vi "Debug.vi"(11 "Msg In":string) -> (3 "Array - String":string[](array[string]))   [LabVIEW 2014, in "Controller.lvlib" / "Controller.lvclass"]
uses:
  Controller.lvclass
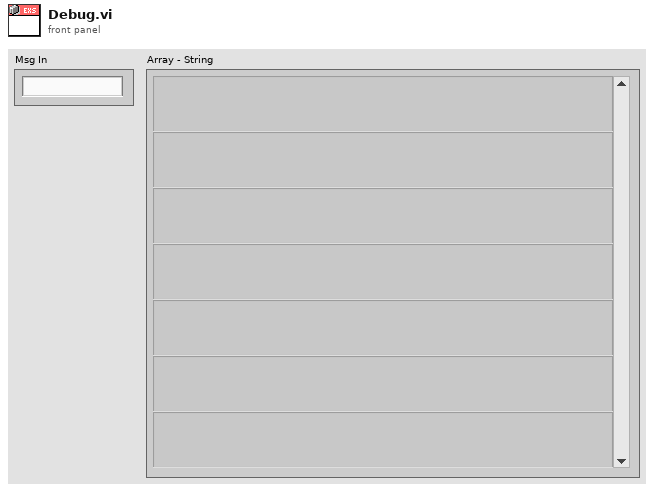
[diagram p1: front panel]
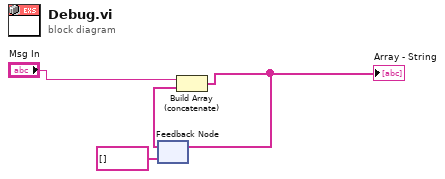
[diagram p0: block diagram]
diagram:
  n1 = feedback #1(string[] []) -> (w2:string[])
  n2 = Build Array (concatenate)("Msg In", w2) -> (w3:string[])
  "Array - String" <- w3
  n3 = feedback-in #1(w3) -> ()
